vi "Dark Current Test MAIN (Brute Force Version).vi"() -> ()   [LabVIEW 2020]
uses:
  <vilib>/DAQmx/create/channels.llb/DAQmx Create Channel (DO-Digital Output).vi
panel:
  in  "Power Supply \nAddress":refnum<visa-resource-name>
  in  "Barcodes in 4":string[](array[string])
  in  "Barcodes in 3":string[](array[string])
  in  "Barcodes in 2":string[](array[string])
  in  "Barcodes in":string[](array[string])
  out "Individual Tube \nCurrent (Nano Amps)":dbl[](array[numeric])
  out "Test Is Running (Red)\nTest Is Stopped (Green)":bool
  in  "Start":bool
  out "Failed Tubes":string[](array[string])
  out "Actual Voltage Level (V)":dbl format="%#_13g"
  out "Power Supply Trip":bool
  out "Actual Current Limit (nA)":dbl format="%#_13g"
  out "Mesurnment Iteration":i32
  in  "stop":bool
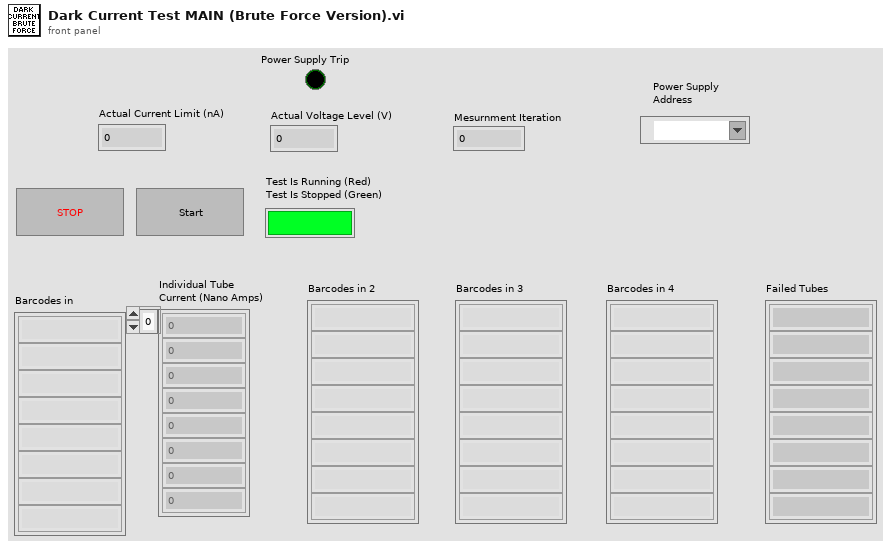
[diagram p1: front panel]
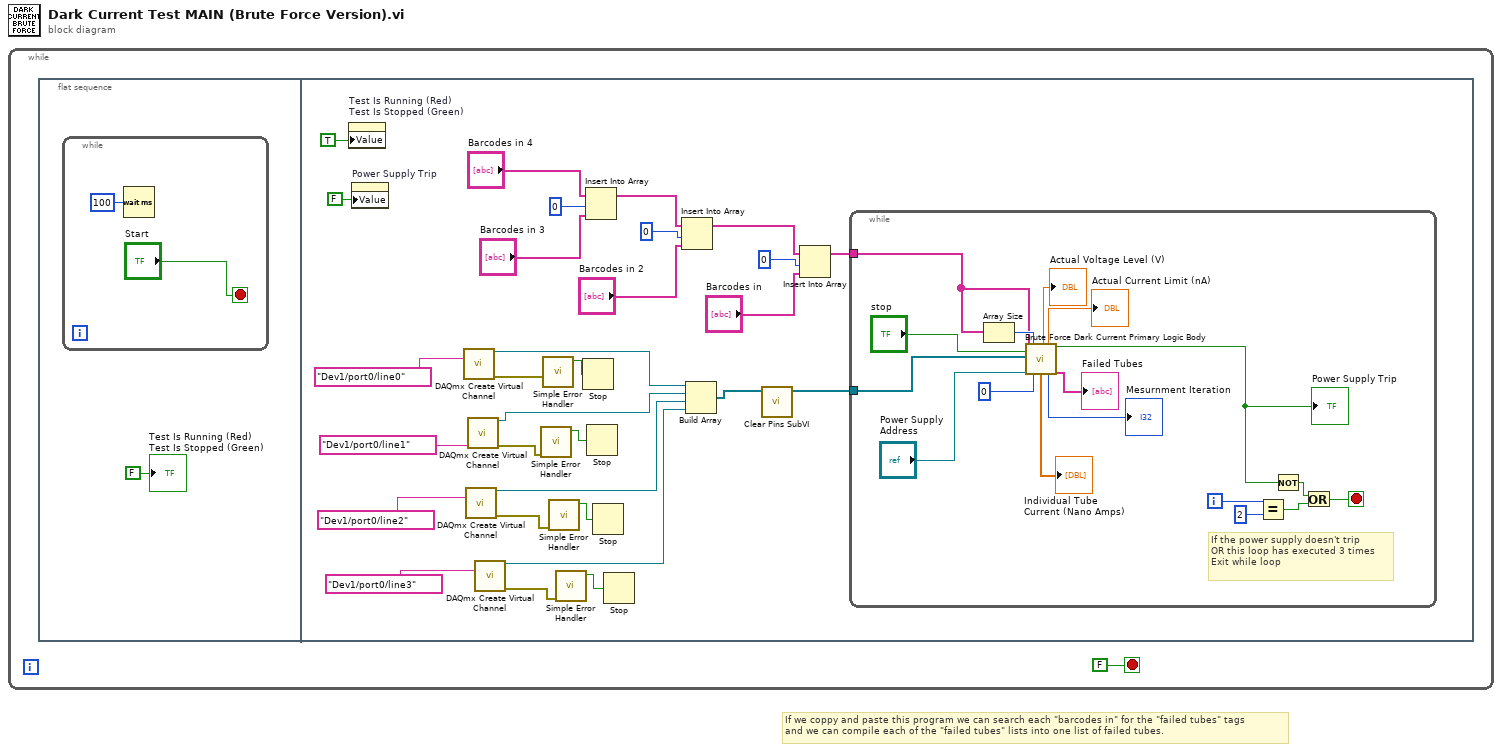
[diagram p0: block diagram]
diagram:
  # "If we coppy and paste this program we can search each \"barcodes in\" for the \"failed tubes\" tags\nand we can compile each of the \"failed tubes\" lists into one list of failed tubes."
  n1 = while {
    stop <- FALSE stop-if-true
    n2 = flat-sequence {
      frame #0 {
        n3 = while {
          stop <- "Start" stop-if-true
          n4 = Wait (ms)(milliseconds to wait=u32 100) -> ()  [unwired: 1 out]
        }
        "Test Is Running (Red)\nTest Is Stopped (Green)" <- FALSE ("Start LED")
      }
      frame #1 {
        n5 = property on="Test Is Running (Red)\nTest Is Stopped (Green)" class="Bool (strict)"("Value"=TRUE) -> ()  [unwired: 2 in, 2 out]
        n6 = property on="Power Supply Trip" class="Bool (strict)"("Value"=FALSE ("Power Supply Trip")) -> ()  [unwired: 2 in, 2 out]
        n7 = call-poly <vilib>:"DAQmx Create Virtual Channel.vi"("lines"=tag "Dev1/port0/line0" ("Data Pin")) -> ("task out"=w20:refnum<k21>, "error out"=w30:errorcluster)  [unwired: 13 in]
        n8 = call-poly <vilib>:"DAQmx Create Virtual Channel.vi"("lines"=tag "Dev1/port0/line2" ("Write Pin")) -> ("task out"=w18:refnum<k21>, "error out"=w28:errorcluster)  [unwired: 13 in]
        n9 = call-poly <vilib>:"DAQmx Create Virtual Channel.vi"("lines"=tag "Dev1/port0/line1" ("Sync Pin")) -> ("task out"=w19:refnum<k21>, "error out"=w29:errorcluster)  [unwired: 13 in]
        n10 = call-poly <vilib>:"DAQmx Create Virtual Channel.vi"("lines"=tag "Dev1/port0/line3" ("Clear Pin")) -> ("task out"=w17:refnum<k21>, "error out"=w27:errorcluster)  [unwired: 13 in]
        n11 = call <vilib>:"Simple Error Handler.vi"("error in (no error)"=w29) -> ("error?"=w23:bool)  [unwired: 4 in, 4 out]
        n12 = call <vilib>:"Simple Error Handler.vi"("error in (no error)"=w30) -> ("error?"=w26:bool)  [unwired: 4 in, 4 out]
        n13 = call <vilib>:"Simple Error Handler.vi"("error in (no error)"=w28) -> ("error?"=w24:bool)  [unwired: 4 in, 4 out]
        n14 = call <vilib>:"Simple Error Handler.vi"("error in (no error)"=w27) -> ("error?"=w25:bool)  [unwired: 4 in, 4 out]
        n15 = Stop(stop? (T)=w26) -> ()
        n16 = Insert Into Array(array="Barcodes in 4", index=0, new element="Barcodes in 3") -> (w12:string[])
        n17 = Stop(stop? (T)=w23) -> ()
        n18 = Stop(stop? (T)=w24) -> ()
        n19 = Stop(stop? (T)=w25) -> ()
        n20 = Insert Into Array(array=w12, index=0, new element="Barcodes in 2") -> (w8:string[])
        n21 = Build Array(w20, w19, w18, w17) -> (w6:refnum<k21>[])
        n22 = call "Clear Pins SubVI.vi"("Pins In"=w6) -> ("Pins Out"=w5:refnum<k21>[])  [unwired: 10 in]
        n23 = Insert Into Array(array=w8, index=0, new element="Barcodes in") -> (w7:string[])
        n24 = while {
          tunnel: w5 -> [w43]
          tunnel: w7 -> [w37]
          i -> [w40]
          stop <- w36 stop-if-true
          # "If the power supply doesn't trip\nOR this loop has executed 3 times Exit while loop"
          n25 = Array Size(array=w37) -> (size(s)=w50:i32)
          n26 = call "Brute Force Dark Current Primary Logic Body.vi"("Barcodes in"=w37, "stop"="stop", "Pins In"=w43, "VISA Refnum in"="Power Supply \nAddress", "Number of Tubes"=w50, "Channel #"=0) -> ("Actual Voltage Level (V)"=→"Actual Voltage Level (V)":dbl, "Individual Tube Current (Nano Amps)"=→"Individual Tube \nCurrent (Nano Amps)":dbl[], "Actual Current Limit (nA)"=→"Actual Current Limit (nA)":dbl, "Mesurnment Iteration"=→"Mesurnment Iteration":i32, "Power Supply Trip"=w41:bool, "Failed Tubes"=→"Failed Tubes":string[])  [unwired: 7 in, 1 out]
          "Power Supply Trip" <- w41
          n27 = Equal?(x=w40, y=2) -> (x = y?=w38:bool)
          n28 = Not(x=w41) -> (.not. x?=w42:bool)
          n29 = Or(x=w42, y=w38) -> (x .or. y?=w36:bool)
        }
      }
    }
  }
